vi "Test Tokenizer Command Types.vi"(8 "error in (no error)":errorcluster) -> (0 "error out":errorcluster)   [LabVIEW 2019]
uses:
  PathTokenizer/PathTokenizer.lvclass
  PathTokenizer/PathTokenizer.lvclass/PathTokenizer.ctl
  <vilib>/addons/_JKI Toolkits/Caraya/classes/Assert/Assert Equal Value_Variant.vi
  <vilib>/addons/_JKI Toolkits/Caraya/classes/Test/Test.lvclass
  <vilib>/addons/_JKI Toolkits/Caraya/classes/Assert/Assert.lvclass
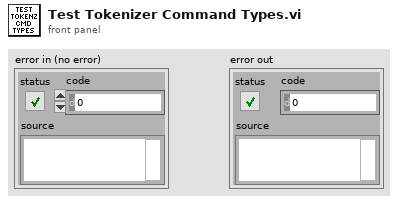
[diagram p1: front panel]
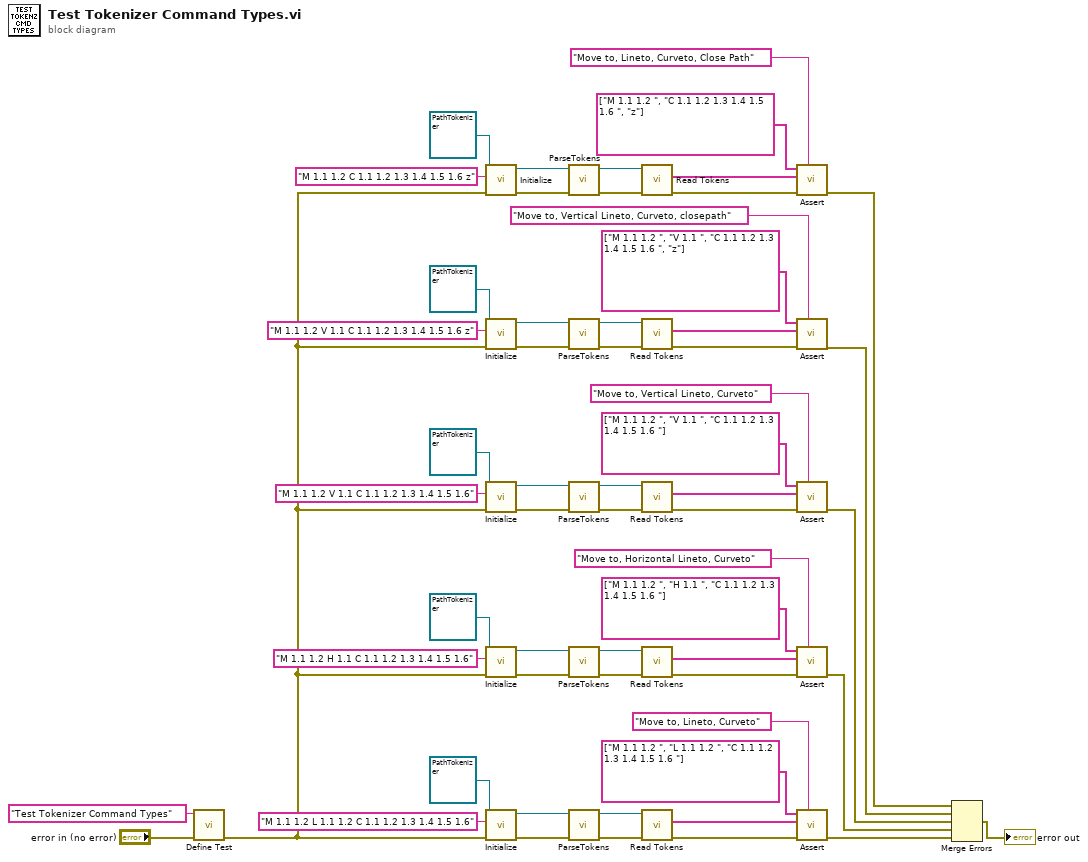
[diagram p0: block diagram]
diagram:
  n1 = call <vilib>:"Define Test.vi"("error in (no error)"="error in (no error)", "Label (VI Title)"="Test Tokenizer Command Types") -> ("error out"=w1:errorcluster)  [unwired: 8 in, 1 out]
  n2 = call "Initialize.vi"("error in (no error)"=w1, "Path Command Text"="M 1.1 1.2 C 1.1 1.2 1.3 1.4 1.5 1.6 z", "PathTokenizer in"=refnum<class "PathTokenizer.lvclass"> refnum) -> ("error out"=w5:errorcluster, "PathTokenizer out"=w6:refnum<class "PathTokenizer.lvclass">)  [unwired: 7 in]
  n3 = call "Initialize.vi"("error in (no error)"=w1, "Path Command Text"="M 1.1 1.2 V 1.1 C 1.1 1.2 1.3 1.4 1.5 1.6 z", "PathTokenizer in"=refnum<class "PathTokenizer.lvclass"> refnum) -> ("error out"=w16:errorcluster, "PathTokenizer out"=w17:refnum<class "PathTokenizer.lvclass">)  [unwired: 7 in]
  n4 = call "Initialize.vi"("error in (no error)"=w1, "Path Command Text"="M 1.1 1.2 V 1.1 C 1.1 1.2 1.3 1.4 1.5 1.6", "PathTokenizer in"=refnum<class "PathTokenizer.lvclass"> refnum) -> ("error out"=w32:errorcluster, "PathTokenizer out"=w31:refnum<class "PathTokenizer.lvclass">)  [unwired: 7 in]
  n5 = call "Initialize.vi"("error in (no error)"=w1, "Path Command Text"="M 1.1 1.2 H 1.1 C 1.1 1.2 1.3 1.4 1.5 1.6", "PathTokenizer in"=refnum<class "PathTokenizer.lvclass"> refnum) -> ("error out"=w38:errorcluster, "PathTokenizer out"=w39:refnum<class "PathTokenizer.lvclass">)  [unwired: 7 in]
  n6 = call "Initialize.vi"("error in (no error)"=w1, "Path Command Text"="M 1.1 1.2 L 1.1 1.2 C 1.1 1.2 1.3 1.4 1.5 1.6", "PathTokenizer in"=refnum<class "PathTokenizer.lvclass"> refnum) -> ("error out"=w54:errorcluster, "PathTokenizer out"=w53:refnum<class "PathTokenizer.lvclass">)  [unwired: 7 in]
  n7 = call "ParseTokens.vi"("error in (no error)"=w5, "PathTokenizer in"=w6) -> ("error out"=w10:errorcluster, "PathTokenizer out"=w9:refnum<class "PathTokenizer.lvclass">)  [unwired: 8 in]
  n8 = call "ParseTokens.vi"("error in (no error)"=w16, "PathTokenizer in"=w17) -> ("error out"=w21:errorcluster, "PathTokenizer out"=w20:refnum<class "PathTokenizer.lvclass">)  [unwired: 8 in]
  n9 = call "ParseTokens.vi"("error in (no error)"=w32, "PathTokenizer in"=w31) -> ("error out"=w27:errorcluster, "PathTokenizer out"=w28:refnum<class "PathTokenizer.lvclass">)  [unwired: 8 in]
  n10 = call "ParseTokens.vi"("error in (no error)"=w38, "PathTokenizer in"=w39) -> ("error out"=w43:errorcluster, "PathTokenizer out"=w42:refnum<class "PathTokenizer.lvclass">)  [unwired: 8 in]
  n11 = call "ParseTokens.vi"("error in (no error)"=w54, "PathTokenizer in"=w53) -> ("error out"=w49:errorcluster, "PathTokenizer out"=w50:refnum<class "PathTokenizer.lvclass">)  [unwired: 8 in]
  n12 = call "Read Tokens.vi"("error in (no error)"=w10, "PathTokenizer in"=w9) -> ("error out"=w12:errorcluster, "Tokens"=w11:string[])  [unwired: 7 in, 1 out]
  n13 = call "Read Tokens.vi"("error in (no error)"=w21, "PathTokenizer in"=w20) -> ("error out"=w23:errorcluster, "Tokens"=w22:string[])  [unwired: 7 in, 1 out]
  n14 = call "Read Tokens.vi"("error in (no error)"=w27, "PathTokenizer in"=w28) -> ("error out"=w25:errorcluster, "Tokens"=w26:string[])  [unwired: 7 in, 1 out]
  n15 = call "Read Tokens.vi"("error in (no error)"=w43, "PathTokenizer in"=w42) -> ("error out"=w45:errorcluster, "Tokens"=w44:string[])  [unwired: 7 in, 1 out]
  n16 = call "Read Tokens.vi"("error in (no error)"=w49, "PathTokenizer in"=w50) -> ("error out"=w47:errorcluster, "Tokens"=w48:string[])  [unwired: 7 in, 1 out]
  n17 = call-poly <vilib>:"Assert.vi"("Label"="Move to, Lineto, Curveto, Close Path", "error in (no error)"=w12, "Y"=w11, "X"=string[] ["M 1.1 1.2 ", "C 1.1 1.2 1.3 1.4 1.5 1.6 ", "z"] ("Tokens")) -> ("error out"=w2:errorcluster)  [unwired: 6 in, 1 out]
  n18 = call-poly <vilib>:"Assert.vi"("Label"="Move to, Vertical Lineto, Curveto, closepath", "error in (no error)"=w23, "Y"=w22, "X"=string[] ["M 1.1 1.2 ", "V 1.1 ", "C 1.1 1.2 1.3 1.4 1.5 1.6 ", "z"] ("Tokens")) -> ("error out"=w13:errorcluster)  [unwired: 6 in, 1 out]
  n19 = call-poly <vilib>:"Assert.vi"("Label"="Move to, Vertical Lineto, Curveto", "error in (no error)"=w25, "Y"=w26, "X"=string[] ["M 1.1 1.2 ", "V 1.1 ", "C 1.1 1.2 1.3 1.4 1.5 1.6 "] ("Tokens")) -> ("error out"=w24:errorcluster)  [unwired: 6 in, 1 out]
  n20 = call-poly <vilib>:"Assert.vi"("Label"="Move to, Horizontal Lineto, Curveto", "error in (no error)"=w45, "Y"=w44, "X"=string[] ["M 1.1 1.2 ", "H 1.1 ", "C 1.1 1.2 1.3 1.4 1.5 1.6 "] ("Tokens")) -> ("error out"=w35:errorcluster)  [unwired: 6 in, 1 out]
  n21 = call-poly <vilib>:"Assert.vi"("Label"="Move to, Lineto, Curveto", "error in (no error)"=w47, "Y"=w48, "X"=string[] ["M 1.1 1.2 ", "L 1.1 1.2 ", "C 1.1 1.2 1.3 1.4 1.5 1.6 "] ("Tokens")) -> ("error out"=w46:errorcluster)  [unwired: 6 in, 1 out]
  n22 = Merge Errors(w2, w13, w24, w35, w46) -> (→"error out":errorcluster)
